vi "Create Transport DAT File.vi"(6 "append to existing file?\n(new file:F)":bool, 8 "error in (no error)":errorcluster, 10 "Wavenames":string[](array[string]), 11 "Control Experiment in":refnum<class "Control Experiment SM.lvclass">) -> (0 "error out":errorcluster, 3 "Control Experiment out":refnum<class "Control Experiment SM.lvclass">)   [LabVIEW 2016, in "Control Experiment SM.lvclass"]
uses:
  Control Experiment SM/Control Experiment SM.lvclass
  <userlib>/LevyLab/LV to ITX/Data/Typedefs/Dictionary--cluster.ctl
  <userlib>/LevyLab/LV to ITX/Data/Data.lvclass
  <userlib>/LevyLab/LV to ITX/Data/Typedefs/File Type--enum.ctl
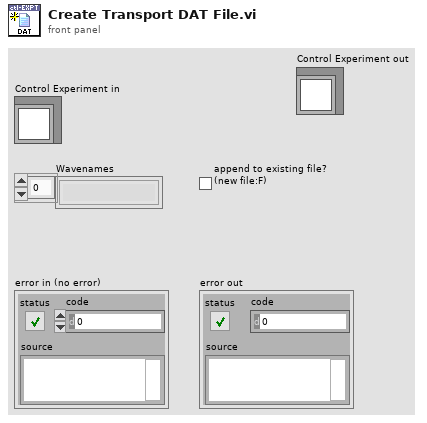
[diagram p1: front panel]
types:
  T1 = typedef "Data.lvclass/File Type--enum.ctl" = enum16{"DAT", "ITX", "TDMS", "VI"}
  T2 = typedef "Data.lvclass/Dictionary--cluster.ctl" = cluster{"key":string, "value":variant}
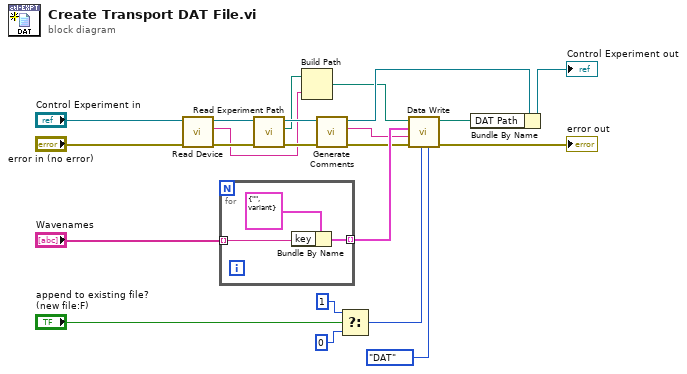
[diagram p0: block diagram]
diagram:
  n1 = call "Read Device.vi"("error in (no error)"="error in (no error)", "Control Experiment in"="Control Experiment in") -> ("error out"=w20:errorcluster, "Device"=w10:string, "Control Experiment out"=w17:refnum<class "Control Experiment SM.lvclass">)  [unwired: 7 in]
  n2 = for {
    tunnel: "Wavenames" -> [w24] mode=indexing
    tunnel: [w23] -> w13 mode=indexing
    n3 = Bundle By Name(cluster=T2 {"key"="", "value"=variant} ("key-value"), "key"=w24) -> (w23:T2)
  }
  n4 = call "Read Experiment Path.vi"("error in (no error)"=w20, "Control Experiment in"=w17) -> ("error out"=w19:errorcluster, "Experiment Path"=w11:path, "Control Experiment out"=w18:refnum<class "Control Experiment SM.lvclass">)  [unwired: 7 in]
  n5 = Build Path(base path=w11, name or relative path=w10) -> (appended path=w2:path)
  n6 = call "Generate Comments.vi"("error in (no error)"=w19, "Control Experiment"=w18) -> ("error out"=w8:errorcluster, "Comments"=w9:string, "Control Experiment out"=w16:refnum<class "Control Experiment SM.lvclass">)  [unwired: 6 in]
  n7 = Select(t=1 ("Append Index"), s="append to existing file?\n(new file:F)", f=0 ("Append Index")) -> (s? t:f=w3:i32)
  n8 = call <userlib>:"Data Write.vi"("File Type"=File_Type--enum."DAT", "Append Index"=w3, "error in (no error)"=w8, "Notes"=w9, "Data (Dictionary)"=w13, "path"=w2) -> ("error out"=→"error out":errorcluster, "path out"=w14:path)  [unwired: 4 in]
  n9 = Bundle By Name(cluster=w16, "DAT Path"=w14) -> (→"Control Experiment out":refnum<class "Control Experiment SM.lvclass">)
